vi "Core Based Monitor Transmit and Receive Messages.vi"() -> ()   [LabVIEW 2019]
doc: "This program opens the specified card, finds the first compatible core, builds a transmit schedule using transmit interval information, and creates filters for two receive messages. It also enables the Sequential Monitor to record transmitted and received messages."
uses:
  <instrlib>/BTI429Lib/Public/Controls/429 Record.ctl
  <instrlib>/BTICardLib/Private/Initialize By Card Number and Core Number.vi
  <instrlib>/BTICardLib/Private/Configure Core From XML.vi
  <instrlib>/BTI429Lib/Private/Tx/Configure/Configure Tx Channel From XML.vi
  <instrlib>/BTI429Lib/Private/Rx/Configure/Configure Rx Channel From XML.vi
  <instrlib>/BTI429Lib/Private/Core/Action-Status/Start All Channels.vi
  <instrlib>/BTI429Lib/Private/Core/Action-Status/Stop All Channels.vi
  <instrlib>/BTICardLib/BTICardLV.lvlib
  <instrlib>/BTI429Lib/BTI429LV.lvlib
panel:
  out "rx channel number":i32
  out "tx channel number":i32
  out "core number":i32
  in  "Rx Channel XML Configuration File":string="Rx Channel Config.xml"
  in  "Tx Channel XML Configuration File":string="Tx Channel Config.xml"
  out "record out":T1 {"type" format="%04x"; "timestamp" format="%08x"; "msgact" format="%04x"; "data" format="%08x"; "timestamph" format="%08x"}
  in  "Core Configuration File":string="Core Config.xml"
  in  "stop":bool
  out "error out":errorcluster
  in  "Card Number":i32
  # "ARINC 429: Core Based Monitor Transmit and Receive Messages"
  # "©2019 Astronics Ballard Technology"
  # "This program opens the specified card, finds the first compatible core, builds a transmit schedule using transmit interval information, and creates filters for two receive messages.  It also enables the Sequential Monitor to record transmitted and received messages. The Core-Based monitor mode is used by selecting perChannelStreaming = false in the Core.XML and using the BTICard monitor functions instead of the BTI429 monitor functions."
  # "Always Stop the card\nand Close the card when\ndone. Otherwise, the hardware\ncontinues to operate."
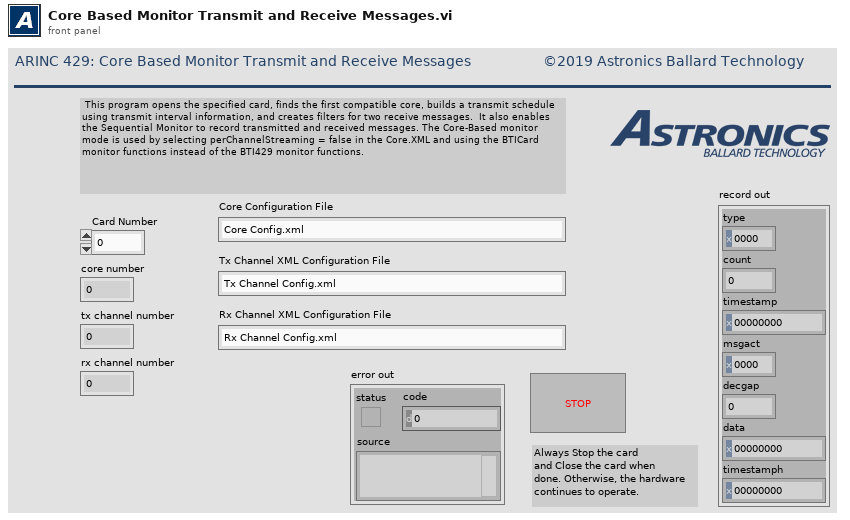
[diagram p1: front panel]
types:
  T1 = typedef "BTI429LV.lvlib/429 Record.ctl" = cluster{"type":u16, "count":u16, "timestamp":u32, "msgact":u16, "decgap":u16, "data":u32, "timestamph":u32}
  T2 = typedef "BTICardLV.lvlib/429 Record.ctl" = cluster{"type":u16, "count":u16, "timestamp":u32, "msgact":u16, "decgap":u16, "data":u32, "timestamph":u32}
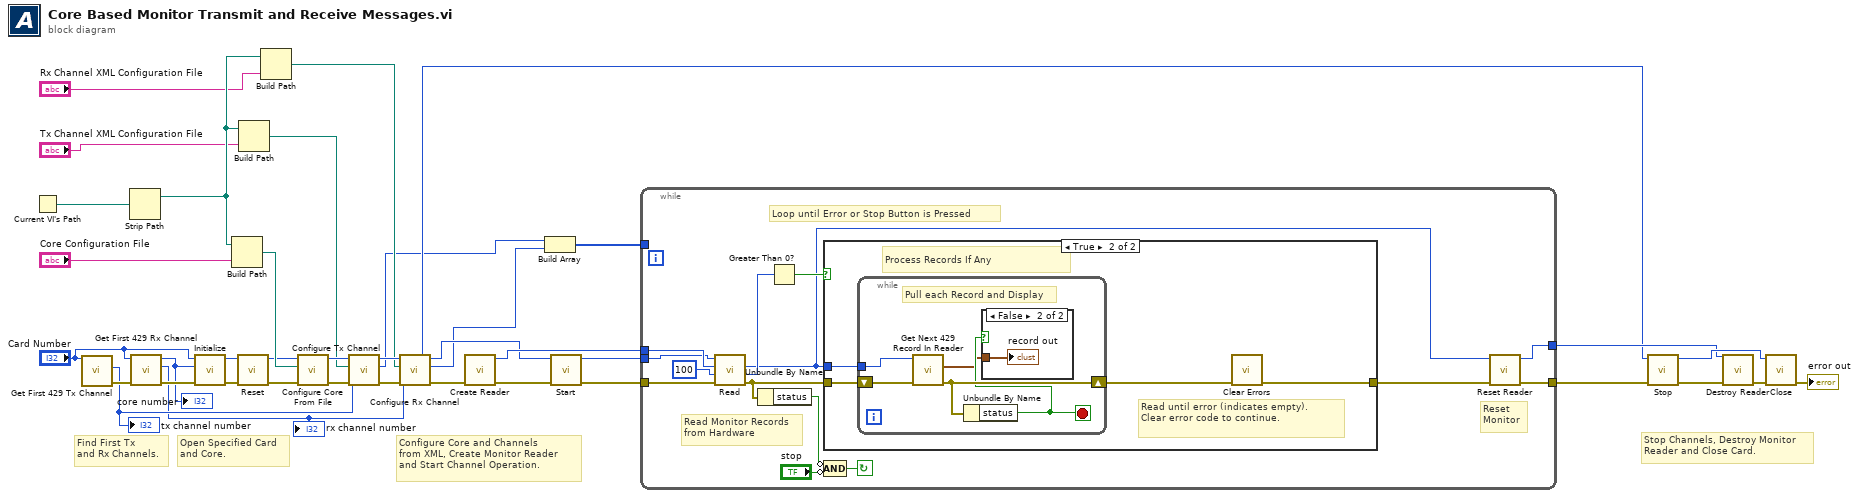
[diagram p0: block diagram]
diagram:
  # "Find First Tx \nand Rx Channels."
  # "Stop Channels, Destroy Monitor\nReader and Close Card."
  # "Configure Core and Channels \nfrom XML, Create Monitor Reader \nand Start Channel Operation."
  # "Open Specified Card\nand Core."
  n1 = Current VI's Path() -> (path=w33:path)
  n2 = call "Get First 429 Tx Channel.vi"("Card Number"="Card Number") -> ("error out"=w10:errorcluster, "Channel Number"=w7:i32)  [unwired: 8 in, 1 out]
  "tx channel number" <- w7
  n3 = Strip Path(path=w33) -> (stripped path=w21:path)  [unwired: 1 out]
  n4 = call "Get First 429 Rx Channel.vi"("error in (no error)"=w10, "Card Number"="Card Number") -> ("error out"=w9:errorcluster, "Channel Number"=w6:i32, "Core Number"=w5:i32)  [unwired: 7 in]
  "core number" <- w5
  "rx channel number" <- w6
  n5 = call-poly <instrlib>:"Initialize.vi"("error in (no error)"=w9, "core number"=w5, "card number"="Card Number") -> ("error out"=w23:errorcluster, "core handle out"=w24:u64)  [unwired: 7 in]
  n6 = Build Path(base path=w21, name or relative path="Core Configuration File") -> (appended path=w32:path)
  n7 = call <instrlib>:"Reset.vi"("error in (no error)"=w23, "core handle in"=w24) -> ("error out"=w25:errorcluster, "core handle out"=w22:u64)  [unwired: 8 in]
  n8 = Build Path(base path=w21, name or relative path="Tx Channel XML Configuration File") -> (appended path=w12:path)
  n9 = Build Path(base path=w21, name or relative path="Rx Channel XML Configuration File") -> (appended path=w11:path)
  n10 = call-poly <instrlib>:"Configure Core From File.vi"("error in (no error)"=w25, "configuration file path"=w32, "core handle in"=w22) -> ("error out"=w18:errorcluster, "core handle out"=w15:u64)  [unwired: 7 in]
  n11 = call-poly <instrlib>:"Configure Tx Channel.vi"("error in (no error)"=w18, "channel number in"=w7, "configuration file path"=w12, "core handle in"=w15) -> ("error out"=w17:errorcluster, "channel handle out"=w4:u64, "core handle out"=w14:u64)  [unwired: 5 in]
  n12 = call-poly <instrlib>:"Configure Rx Channel.vi"("error in (no error)"=w17, "channel number in"=w6, "configuration file path"=w11, "core handle in"=w14) -> ("error out"=w16:errorcluster, "channel handle out"=w3:u64, "core handle out"=w13:u64)  [unwired: 5 in]
  n13 = call <instrlib>:"Create Reader.vi"("error in (no error)"=w16) -> ("error out"=w30:errorcluster, "core reader handle out"=w34:u64)  [unwired: 9 in]
  n14 = Build Array(w4, w3) -> (w2:u64[])
  n15 = call-poly <instrlib>:"Start.vi"("error in (no error)"=w30, "core handle in"=w13) -> ("error out"=w35:errorcluster, "core handle out"=w1:u64)  [unwired: 8 in]
  n16 = while {
    tunnel: [w43] -> w36
    tunnel: w34 -> [w48]
    tunnel: w35 -> [w49]
    tunnel: [w39] -> w26
    tunnel: w2 -> [_]
    tunnel: w1 -> [w38]
    stop <- w50 continue-if-true
    # "Reset\nMonitor"
    # "Read Monitor Records\nfrom Hardware"
    # "Loop until Error or Stop Button is Pressed"
    n17 = call <instrlib>:"Read.vi"("error in (no error)"=w49, "max bytes to read"=100 ("max records to read"), "core reader handle in"=w48, "core handle in"=w38) -> ("error out"=w41:errorcluster, "bytes read"=w44:i32, "core reader handle out"=w42:u64)  [unwired: 4 in, 1 out]
    n18 = Unbundle By Name(w41) -> ("status"=w51:bool)
    n19 = Greater Than 0?(x=w44) -> (x > 0?=w45:bool)
    n20 = case shown="True" w45 {
      tunnel: w42 -> [_ w56]
      tunnel: w41 -> [w52 w55]
      tunnel: [w52 w53] -> w40
      frame False {
      }
      frame True {
        # "Read until error (indicates empty).\nClear error code to continue."
        # "Process Records If Any"
        n21 = while {
          tunnel: w56 -> [w61]
          shift-right: [w59] -> w54
          shift-left: w55 -> [w60]
          stop <- w58 stop-if-true
          # "Pull each Record and Display"
          n22 = call <instrlib>:"Get Next 429 Record In Reader.vi"("error in (no error)"=w60, "core reader handle in"=w61) -> ("error out"=w59:errorcluster, "record out"=w57:T2)  [unwired: 7 in, 1 out]
          n23 = Unbundle By Name(w59) -> ("status"=w58:bool)
          n24 = case shown="False" w58 {
            tunnel: w57 -> [_ w62]
            frame True {
            }
            frame False {
              "record out" <- w62
            }
          }
        }
        n25 = call <vilib>:"Clear Errors.vi"("error in (no error)"=w54) -> ("error out"=w53:errorcluster)  [unwired: 5 in, 1 out]
      }
    }
    n26 = Compound Arithmetic op=AND(invert w51, invert "stop") -> (w50:bool)
    n27 = call <instrlib>:"Reset Reader.vi"("error in (no error)"=w40, "reader handle in"=w42) -> ("error out"=w43:errorcluster, "reader handle out"=w39:u64)  [unwired: 8 in]
  }
  n28 = call-poly <instrlib>:"Stop.vi"("error in (no error)"=w36, "core handle in"=w22) -> ("error out"=w29:errorcluster, "core handle out"=w27:u64)  [unwired: 8 in]
  n29 = call <instrlib>:"Destroy Reader.vi"("error in (no error)"=w29, "reader handle in"=w26) -> ("error out"=w28:errorcluster)  [unwired: 9 in]
  n30 = call <instrlib>:"Close.vi"("error in (no error)"=w28, "core handle in"=w27) -> ("error out"=→"error out":errorcluster)  [unwired: 8 in, 1 out]
